vi "ledtest2.vi"() -> ()   [LabVIEW 2012]
panel:
  out "Total number of pulses sent":u64
  in  "stop":bool
  out "Randomly generated testpulse separation out":u32
  out "Is Test Pulse?":bool
  in  "Testpulse Time Delay (20 ns ticks)":u32=14
  in  "Testpulse duration (20 ns ticks)":u32=5
  in  "Testpulser On/Off":bool
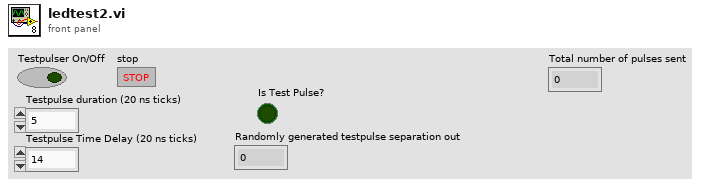
[diagram p1: front panel]
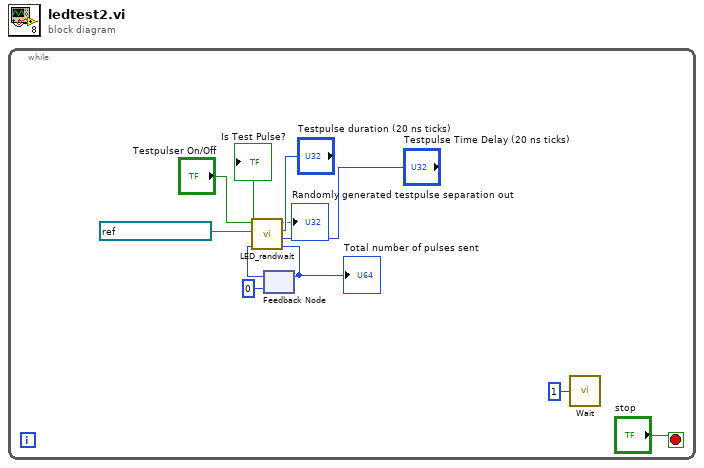
[diagram p0: block diagram]
diagram:
  n1 = while {
    stop <- "stop" stop-if-true
    n2 = feedback #1(u64 0 ("Total number of pulses sent")) -> (w7:u64)
    n3 = call "LED_randwait.vi"("FPGA I/O In"=refnum<k21> "IO Module\\D0 0", "seed"=w7, "Testpulse Time Delay (20 ns ticks)"="Testpulse Time Delay (20 ns ticks)", "Testpulse duration (20 ns ticks)"="Testpulse duration (20 ns ticks)", "Testpulser On/Off"="Testpulser On/Off") -> ("Total number of pulses sent"=w6:u64, 3:→"Randomly generated testpulse separation out", "Is Test Pulse?"=→"Is Test Pulse?":bool)  [unwired: 4 in]
    "Total number of pulses sent" <- w6
    n4 = feedback-in #1(w6) -> ()
    n5 = call "Wait"("Count(mSec)"=u32 1) -> ()  [unwired: 1 out]
  }
